vi "SubVI_Save_Optimal_Model.vi"(4 "Training_settings":string, 6 "Optimum Window Size":i32, 7 "Number of Trials":i32, 8 "error in (no error)":errorcluster, 9 "Hyperparameters":T1, 10 "Go Epochs in":dbl[][](array[numeric]), 11 "Best (Metric)":dbl) -> (0 "error out":errorcluster, 3 "Case to Switch to":i32)   [LabVIEW 2020]
uses:
  Global 1.vi
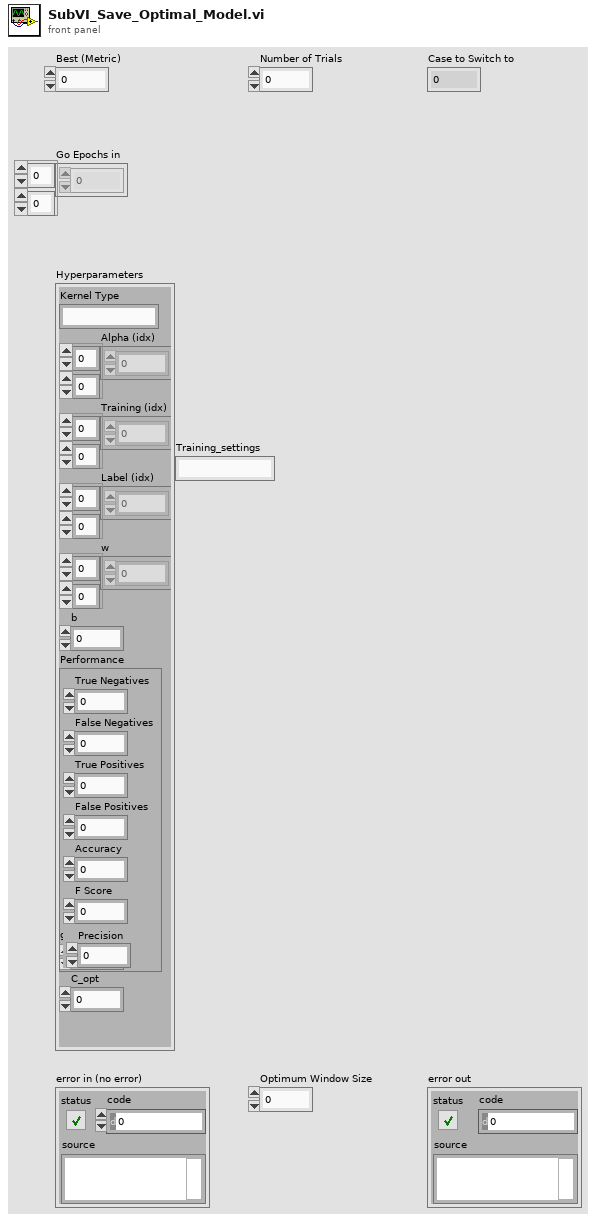
[diagram p1: front panel]
types:
  T1 = cluster{"Kernel Type":string, "Alpha (idx)":dbl[][], "Training (idx)":dbl[][], "Label (idx)":dbl[][], "w":dbl[][], "b":dbl, "Performance":cluster{"True Negatives":i32, "False Negatives":i32, "True Positives":i32, "False Positives":i32, "Accuracy":dbl, "F Score":dbl, "Precision":dbl}, "gamma_opt":dbl, "C_opt":dbl}
  T2 = enum16{"open", "open or create", "create or replace", "create", "open (read-only)"}
  T3 = enum16{"open", "replace", "create", "open or create", "replace or create", "replace or create with confirmation"}
  T4 = cluster{"Hyperparameters":cluster{"Kernel Type":string, "Alpha (idx)":dbl[][], "Training (idx)":dbl[][], "Label (idx)":dbl[][], "w":dbl[][], "b":dbl, "Performance":cluster{"True Negatives":i32, "False Negatives":i32, "True Positives":i32, "False Positives":i32, "Accuracy":dbl, "F Score":dbl, "Precision":dbl}, "gamma_opt":dbl, "C_opt":dbl}, "Optimum Window Size":i32, "Best (Metric)":dbl, dbl[][]}
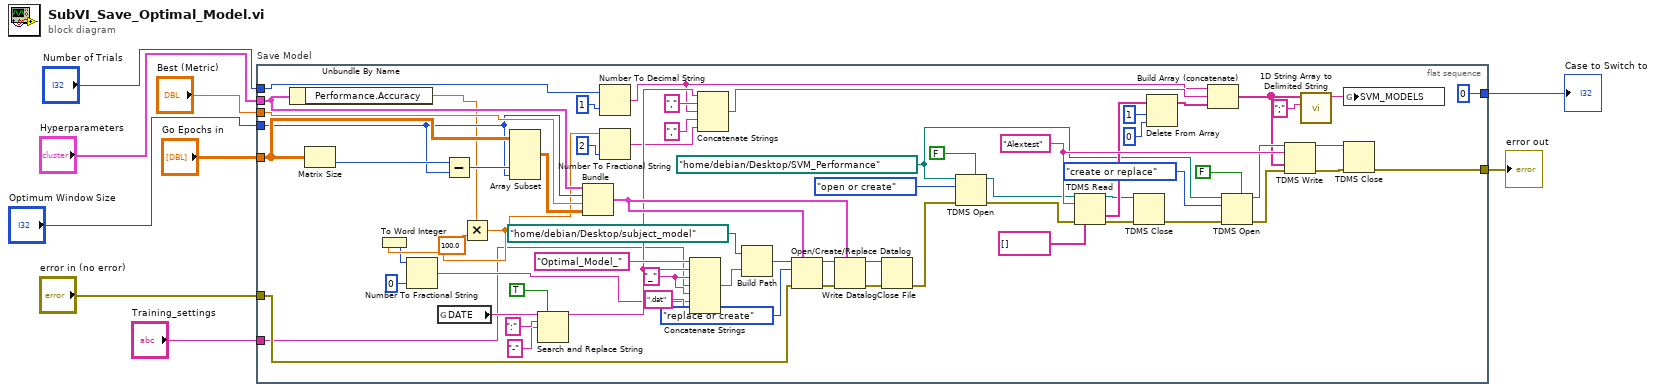
[diagram p0: block diagram]
diagram:
  n1 = flat-sequence "Save Model" {
    tunnel: "Best (Metric)" -> [w75]
    tunnel: "Hyperparameters" -> [w43]
    tunnel: "Go Epochs in" -> [w74]
    tunnel: "Optimum Window Size" -> [w71]
    tunnel: "error in (no error)" -> [w62]
    tunnel: [w41] -> w6
    tunnel: [0 ("Tab Select")] -> w7
    tunnel: "Number of Trials" -> [w20]
    tunnel: "Training_settings" -> [w10]
    frame #0 {
      w11 = "_" ("string")
      w30 = path "/home/debian/Desktop/SVM_Performance" ("base path")
      w49 = "Alextest" ("group name in (Untitled)")
      n2 = Unbundle By Name(w43) -> ("Performance.Accuracy"=w19:dbl)
      n3 = Matrix Size(0:w74) -> (2:w73:i32)  [unwired: 1 out]
      n4 = global read "Global 1.vi" "DATE"() -> (w21:string)
      n5 = Subtract(x=w73, y=w71) -> (x-y=w72:i32)
      n6 = Multiply(x=w19, y=100.0) -> (x*y=w17:dbl)
      n7 = To Word Integer(number=w17) -> (16bit integer=w16:i16)
      n8 = Number To Fractional String(number=w16, precision (6)=i16 0) -> (F-format string=w12:string)  [unwired: 2 in]
      n9 = Array Subset(array=w74, index (col)=w72, length (col)=w71) -> (w70:dbl[][])  [unwired: 2 in]
      n10 = Search and Replace String(replace all?=TRUE ("replace all? (F)"), input string=w21, search string=":" ("input string"), replace string="-" ("replace string (\"\")")) -> (result string=w39:string)  [unwired: 4 in, 3 out]
      n11 = Bundle("Hyperparameters"=w43, "Optimum Window Size"=w71, "Best (Metric)"=w75, w70) -> (w61:T4)  [unwired: 1 in]
      n12 = Number To Decimal String(number=w20, width (-)=i16 1) -> (decimal integer string=w35:string)
      n13 = Number To Fractional String(number=w17, precision (6)=i16 2 ("width (-)")) -> (F-format string=w25:string)  [unwired: 2 in]
      n14 = Concatenate Strings("Optimal_Model_" ("string"), w39, w11, w10, w11, w12, ".dat" ("string")) -> (w56:string)
      n15 = Concatenate Strings(w39, "," ("string"), w35, "," ("string"), w25) -> (w36:string)
      n16 = Build Path(base path=path "/home/debian/Desktop/subject_model", name or relative path=w56) -> (appended path=w64:path)
      n17 = Open/Create/Replace Datalog(5:w61, 8:w62, 10:T3."replace or create" ("operation (0:open)"), 11:w64) -> (0:w65:errorcluster, 3:w68:refnum<k1>)  [unwired: 2 in, 1 out]
      n18 = Write Datalog(4:w65, 6:w61, 7:w68) -> (0:w66:errorcluster, 3:w67:refnum<k1>)
      n19 = Close File(refnum=w67, error in=w66) -> (error out=w42:errorcluster)  [unwired: 1 out]
      n20 = TDMS Open(5:FALSE ("create index file? (T)"), 8:w42, 10:T2."open or create" ("operation (0:open)"), 11:w30) -> (0:w50:errorcluster, 3:w48:refnum<k34>)  [unwired: 3 in]
      n21 = TDMS Read(0:w48, 5:w49, 11:w50, 12:string[] []) -> (4:w31:refnum<k34>, 10:w46:string[], 15:w33:errorcluster)  [unwired: 4 in, 3 out]
      n22 = TDMS Close(8:w33, 11:w31) -> (0:w32:errorcluster)  [unwired: 1 out]
      n23 = Delete From Array(array=w46, length=1, index=0 ("index (row)")) -> (array with subset deleted=w37:string[])  [unwired: 1 out]
      n24 = Build Array (concatenate)(w35, w36, w37) -> (w24:string[])
      n25 = TDMS Open(5:FALSE ("create index file? (T)"), 8:w32, 10:T2."create or replace" ("operation (0:open)"), 11:w30) -> (0:w26:errorcluster, 3:w27:refnum<k34>)  [unwired: 3 in]
      n26 = TDMS Write(0:w27, 5:w49, 9:w24, 11:w26) -> (4:w52:refnum<k34>, 15:w53:errorcluster)  [unwired: 2 in, 2 out]
      n27 = call <vilib>:"1D String Array to Delimited String.vi"("delimiter"=";", "string array"=w24) -> ("delimited string"=w22:string)  [unwired: 9 in]
      n28 = global write "Global 1.vi" "SVM_MODELS"(w22) -> ()
      n29 = TDMS Close(8:w53, 11:w52) -> (0:w41:errorcluster)  [unwired: 1 out]
    }
  }
  "Case to Switch to" <- w7
  "error out" <- w6
